vi "Stop Core.vi"(10 "final error code":i32, 11 "Logger in":refnum<class "Logger.lvclass">) -> (3 "Logger out":refnum<class "Logger.lvclass">)   [LabVIEW 2019, in "Logger.lvlib" / "Logger.lvclass"]
doc: "(<B>Filename</B>: Actor Framework.lvlib:Actor.lvclass:Stop Core.vi)\n\nDefines what the actor does before it stops. Use the <B>final error code</B> input to determine whether the actor shut down in response to an error.\n\nBy default, this method passes the Stop message along to all auto-stop nested actors. A descendant class may override this method to define additional behavior, such as shutting down any processes the actor initiated in its override of the Actor Core method."
uses:
  Logger.lvclass
  <vilib>/ActorFramework/Actor/Actor.lvclass
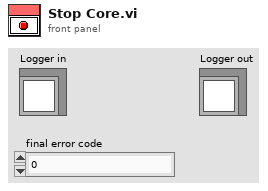
[diagram p1: front panel]
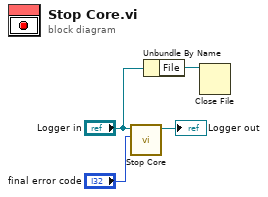
[diagram p0: block diagram]
diagram:
  n1 = call-parent "Stop Core.vi"("final error code"="final error code", "Actor in"="Logger in") -> ("Actor out"=→"Logger out":refnum<class "Logger.lvclass">)  [unwired: 9 in]
  n2 = Unbundle By Name("Logger in") -> ("File"=w1:refnum<file>)
  n3 = Close File(refnum=w1) -> ()  [unwired: 1 in, 2 out]
